vi "PulseDetectAndSwitch60.vi"(9 "Laser bits in":bool[](array[boolean])=[FALSE, FALSE, FALSE, FALSE, FALSE, FALSE, FALSE, FALSE, FALSE, FALSE, FALSE, FALSE, FALSE, FALSE, FALSE, FALSE, FALSE, FALSE, FALSE, FALSE, FALSE, FALSE, FALSE, FALSE, FALSE, FALSE, FALSE, FALSE, FALSE, FALSE, FALSE, FALSE, FALSE, FALSE, FALSE, FALSE, FALSE, FALSE, FALSE, FALSE, FALSE, FALSE, FALSE, FALSE, FALSE, FALSE, FALSE, FALSE, FALSE, FALSE, FALSE, FALSE, FALSE, FALSE, FALSE, FALSE, FALSE, FALSE, FALSE, FALSE], 10 "Last area":bool, 11 "Last laser bit in":bool) -> (1 "Area bits out":bool[](array[boolean]), 2 "New last area out":bool, 3 "New last laser bit out":bool)   [LabVIEW 2012]
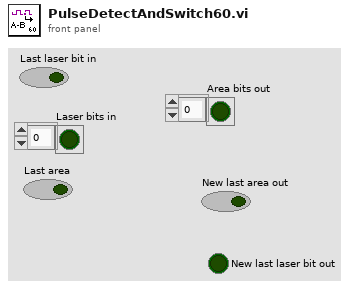
[diagram p1: front panel]
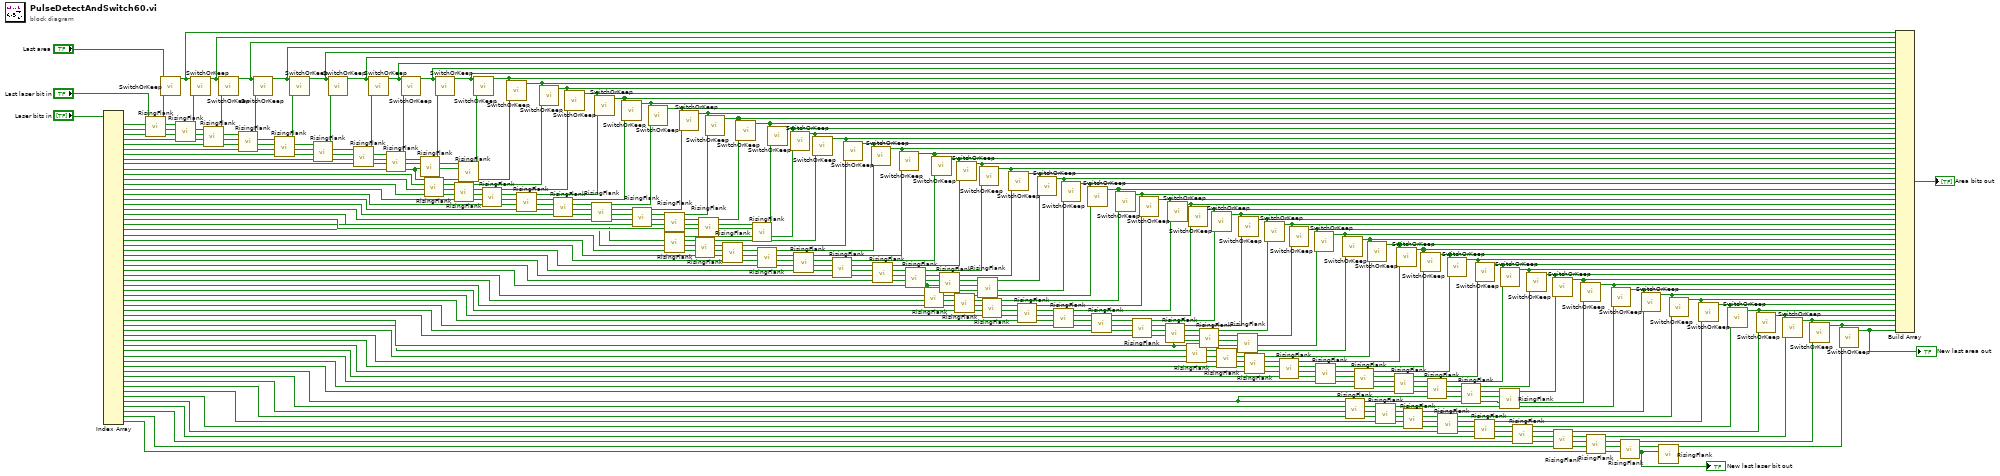
[diagram p0: block diagram]
diagram:
  n1 = Index Array(array="Laser bits in") -> (element #1=w182:bool, element #2=w181:bool, element #3=w180:bool, element #4=w179:bool, element #5=w178:bool, element #6=w177:bool, element #7=w176:bool, element #8=w175:bool, element #9=w174:bool, element #10=w152:bool, element #11=w151:bool, element #12=w150:bool, element #13=w149:bool, element #14=w148:bool, element #15=w147:bool, element #16=w146:bool, element #17=w145:bool, element #18=w144:bool, element #19=w143:bool, element #20=w142:bool, element #21=w141:bool, element #22=w140:bool, element #23=w139:bool, element #24=w138:bool, element #25=w1:bool, element #26=w137:bool, element #27=w136:bool, element #28=w135:bool, element #29=w134:bool, element #30=w133:bool, element #31=w132:bool, element #32=w131:bool, element #33=w130:bool, element #34=w129:bool, element #35=w2:bool, element #36=w128:bool, element #37=w127:bool, element #38=w126:bool, element #39=w125:bool, element #40=w124:bool, element #41=w123:bool, element #42=w3:bool, element #43=w122:bool, element #44=w121:bool, element #45=w120:bool, element #46=w119:bool, element #47=w118:bool, element #48=w4:bool, element #49=w117:bool, element #50=w116:bool, element #51=w115:bool, element #52=w114:bool, element #53=w113:bool, element #54=w112:bool, element #55=w111:bool, element #56=w110:bool, element #57=w109:bool, element #58=w108:bool, element #59=w107:bool, element #60=w106:bool)  [unwired: 60 in]
  "New last laser bit out" <- w106
  n2 = call "RisingFlank.vi"("2nd sample"=w182, "1st sample"="Last laser bit in") -> ("Rising flank?"=w172:bool)  [unwired: 7 in]
  n3 = call "SwitchOrKeep.vi"("Rising flank? in"=w172, "Last state in"="Last area") -> ("New state out"=w162:bool)  [unwired: 9 in]
  n4 = call "RisingFlank.vi"("2nd sample"=w181, "1st sample"=w182) -> ("Rising flank?"=w171:bool)  [unwired: 7 in]
  n5 = call "SwitchOrKeep.vi"("Rising flank? in"=w171, "Last state in"=w162) -> ("New state out"=w161:bool)  [unwired: 9 in]
  n6 = call "RisingFlank.vi"("2nd sample"=w180, "1st sample"=w181) -> ("Rising flank?"=w170:bool)  [unwired: 7 in]
  n7 = call "SwitchOrKeep.vi"("Rising flank? in"=w170, "Last state in"=w161) -> ("New state out"=w160:bool)  [unwired: 9 in]
  n8 = call "RisingFlank.vi"("2nd sample"=w179, "1st sample"=w180) -> ("Rising flank?"=w169:bool)  [unwired: 7 in]
  n9 = call "SwitchOrKeep.vi"("Rising flank? in"=w169, "Last state in"=w160) -> ("New state out"=w159:bool)  [unwired: 9 in]
  n10 = call "RisingFlank.vi"("2nd sample"=w178, "1st sample"=w179) -> ("Rising flank?"=w168:bool)  [unwired: 7 in]
  n11 = call "SwitchOrKeep.vi"("Rising flank? in"=w168, "Last state in"=w159) -> ("New state out"=w158:bool)  [unwired: 9 in]
  n12 = call "RisingFlank.vi"("2nd sample"=w177, "1st sample"=w178) -> ("Rising flank?"=w167:bool)  [unwired: 7 in]
  n13 = call "SwitchOrKeep.vi"("Rising flank? in"=w167, "Last state in"=w158) -> ("New state out"=w157:bool)  [unwired: 9 in]
  n14 = call "RisingFlank.vi"("2nd sample"=w176, "1st sample"=w177) -> ("Rising flank?"=w166:bool)  [unwired: 7 in]
  n15 = call "SwitchOrKeep.vi"("Rising flank? in"=w166, "Last state in"=w157) -> ("New state out"=w156:bool)  [unwired: 9 in]
  n16 = call "RisingFlank.vi"("2nd sample"=w175, "1st sample"=w176) -> ("Rising flank?"=w165:bool)  [unwired: 7 in]
  n17 = call "SwitchOrKeep.vi"("Rising flank? in"=w165, "Last state in"=w156) -> ("New state out"=w155:bool)  [unwired: 9 in]
  n18 = call "RisingFlank.vi"("2nd sample"=w174, "1st sample"=w175) -> ("Rising flank?"=w164:bool)  [unwired: 7 in]
  n19 = call "RisingFlank.vi"("2nd sample"=w151, "1st sample"=w152) -> ("Rising flank?"=w104:bool)  [unwired: 7 in]
  n20 = call "SwitchOrKeep.vi"("Rising flank? in"=w164, "Last state in"=w155) -> ("New state out"=w154:bool)  [unwired: 9 in]
  n21 = call "RisingFlank.vi"("2nd sample"=w150, "1st sample"=w151) -> ("Rising flank?"=w102:bool)  [unwired: 7 in]
  n22 = call "RisingFlank.vi"("2nd sample"=w152, "1st sample"=w174) -> ("Rising flank?"=w163:bool)  [unwired: 7 in]
  n23 = call "SwitchOrKeep.vi"("Rising flank? in"=w163, "Last state in"=w154) -> ("New state out"=w105:bool)  [unwired: 9 in]
  n24 = call "RisingFlank.vi"("2nd sample"=w149, "1st sample"=w150) -> ("Rising flank?"=w100:bool)  [unwired: 7 in]
  n25 = call "SwitchOrKeep.vi"("Rising flank? in"=w104, "Last state in"=w105) -> ("New state out"=w103:bool)  [unwired: 9 in]
  n26 = call "RisingFlank.vi"("2nd sample"=w148, "1st sample"=w149) -> ("Rising flank?"=w98:bool)  [unwired: 7 in]
  n27 = call "SwitchOrKeep.vi"("Rising flank? in"=w102, "Last state in"=w103) -> ("New state out"=w101:bool)  [unwired: 9 in]
  n28 = call "RisingFlank.vi"("2nd sample"=w147, "1st sample"=w148) -> ("Rising flank?"=w96:bool)  [unwired: 7 in]
  n29 = call "SwitchOrKeep.vi"("Rising flank? in"=w100, "Last state in"=w101) -> ("New state out"=w99:bool)  [unwired: 9 in]
  n30 = call "RisingFlank.vi"("2nd sample"=w146, "1st sample"=w147) -> ("Rising flank?"=w94:bool)  [unwired: 7 in]
  n31 = call "SwitchOrKeep.vi"("Rising flank? in"=w98, "Last state in"=w99) -> ("New state out"=w97:bool)  [unwired: 9 in]
  n32 = call "SwitchOrKeep.vi"("Rising flank? in"=w96, "Last state in"=w97) -> ("New state out"=w95:bool)  [unwired: 9 in]
  n33 = call "RisingFlank.vi"("2nd sample"=w145, "1st sample"=w146) -> ("Rising flank?"=w92:bool)  [unwired: 7 in]
  n34 = call "SwitchOrKeep.vi"("Rising flank? in"=w94, "Last state in"=w95) -> ("New state out"=w93:bool)  [unwired: 9 in]
  n35 = call "RisingFlank.vi"("2nd sample"=w144, "1st sample"=w145) -> ("Rising flank?"=w91:bool)  [unwired: 7 in]
  n36 = call "RisingFlank.vi"("2nd sample"=w141, "1st sample"=w142) -> ("Rising flank?"=w84:bool)  [unwired: 7 in]
  n37 = call "SwitchOrKeep.vi"("Rising flank? in"=w92, "Last state in"=w93) -> ("New state out"=w90:bool)  [unwired: 9 in]
  n38 = call "RisingFlank.vi"("2nd sample"=w140, "1st sample"=w141) -> ("Rising flank?"=w82:bool)  [unwired: 7 in]
  n39 = call "RisingFlank.vi"("2nd sample"=w143, "1st sample"=w144) -> ("Rising flank?"=w88:bool)  [unwired: 7 in]
  n40 = call "SwitchOrKeep.vi"("Rising flank? in"=w91, "Last state in"=w90) -> ("New state out"=w89:bool)  [unwired: 9 in]
  n41 = call "RisingFlank.vi"("2nd sample"=w139, "1st sample"=w140) -> ("Rising flank?"=w80:bool)  [unwired: 7 in]
  n42 = call "SwitchOrKeep.vi"("Rising flank? in"=w88, "Last state in"=w89) -> ("New state out"=w87:bool)  [unwired: 9 in]
  n43 = call "RisingFlank.vi"("2nd sample"=w142, "1st sample"=w143) -> ("Rising flank?"=w86:bool)  [unwired: 7 in]
  n44 = call "RisingFlank.vi"("2nd sample"=w138, "1st sample"=w139) -> ("Rising flank?"=w78:bool)  [unwired: 7 in]
  n45 = call "SwitchOrKeep.vi"("Rising flank? in"=w86, "Last state in"=w87) -> ("New state out"=w85:bool)  [unwired: 9 in]
  n46 = call "SwitchOrKeep.vi"("Rising flank? in"=w84, "Last state in"=w85) -> ("New state out"=w83:bool)  [unwired: 9 in]
  n47 = call "RisingFlank.vi"("2nd sample"=w1, "1st sample"=w138) -> ("Rising flank?"=w76:bool)  [unwired: 7 in]
  n48 = call "SwitchOrKeep.vi"("Rising flank? in"=w82, "Last state in"=w83) -> ("New state out"=w81:bool)  [unwired: 9 in]
  n49 = call "RisingFlank.vi"("2nd sample"=w137, "1st sample"=w1) -> ("Rising flank?"=w74:bool)  [unwired: 7 in]
  n50 = call "SwitchOrKeep.vi"("Rising flank? in"=w80, "Last state in"=w81) -> ("New state out"=w79:bool)  [unwired: 9 in]
  n51 = call "SwitchOrKeep.vi"("Rising flank? in"=w78, "Last state in"=w79) -> ("New state out"=w77:bool)  [unwired: 9 in]
  n52 = call "RisingFlank.vi"("2nd sample"=w136, "1st sample"=w137) -> ("Rising flank?"=w72:bool)  [unwired: 7 in]
  n53 = call "SwitchOrKeep.vi"("Rising flank? in"=w76, "Last state in"=w77) -> ("New state out"=w75:bool)  [unwired: 9 in]
  n54 = call "RisingFlank.vi"("2nd sample"=w135, "1st sample"=w136) -> ("Rising flank?"=w70:bool)  [unwired: 7 in]
  n55 = call "RisingFlank.vi"("2nd sample"=w132, "1st sample"=w133) -> ("Rising flank?"=w64:bool)  [unwired: 7 in]
  n56 = call "SwitchOrKeep.vi"("Rising flank? in"=w74, "Last state in"=w75) -> ("New state out"=w73:bool)  [unwired: 9 in]
  n57 = call "RisingFlank.vi"("2nd sample"=w134, "1st sample"=w135) -> ("Rising flank?"=w68:bool)  [unwired: 7 in]
  n58 = call "RisingFlank.vi"("2nd sample"=w131, "1st sample"=w132) -> ("Rising flank?"=w62:bool)  [unwired: 7 in]
  n59 = call "SwitchOrKeep.vi"("Rising flank? in"=w72, "Last state in"=w73) -> ("New state out"=w71:bool)  [unwired: 9 in]
  n60 = call "RisingFlank.vi"("2nd sample"=w133, "1st sample"=w134) -> ("Rising flank?"=w66:bool)  [unwired: 7 in]
  n61 = call "SwitchOrKeep.vi"("Rising flank? in"=w70, "Last state in"=w71) -> ("New state out"=w69:bool)  [unwired: 9 in]
  n62 = call "RisingFlank.vi"("2nd sample"=w130, "1st sample"=w131) -> ("Rising flank?"=w60:bool)  [unwired: 7 in]
  n63 = call "SwitchOrKeep.vi"("Rising flank? in"=w68, "Last state in"=w69) -> ("New state out"=w67:bool)  [unwired: 9 in]
  n64 = call "RisingFlank.vi"("2nd sample"=w129, "1st sample"=w130) -> ("Rising flank?"=w58:bool)  [unwired: 7 in]
  n65 = call "SwitchOrKeep.vi"("Rising flank? in"=w66, "Last state in"=w67) -> ("New state out"=w65:bool)  [unwired: 9 in]
  n66 = call "RisingFlank.vi"("2nd sample"=w2, "1st sample"=w129) -> ("Rising flank?"=w56:bool)  [unwired: 7 in]
  n67 = call "SwitchOrKeep.vi"("Rising flank? in"=w64, "Last state in"=w65) -> ("New state out"=w63:bool)  [unwired: 9 in]
  n68 = call "SwitchOrKeep.vi"("Rising flank? in"=w62, "Last state in"=w63) -> ("New state out"=w61:bool)  [unwired: 9 in]
  n69 = call "RisingFlank.vi"("2nd sample"=w128, "1st sample"=w2) -> ("Rising flank?"=w55:bool)  [unwired: 7 in]
  n70 = call "SwitchOrKeep.vi"("Rising flank? in"=w60, "Last state in"=w61) -> ("New state out"=w59:bool)  [unwired: 9 in]
  n71 = call "RisingFlank.vi"("2nd sample"=w127, "1st sample"=w128) -> ("Rising flank?"=w54:bool)  [unwired: 7 in]
  n72 = call "SwitchOrKeep.vi"("Rising flank? in"=w58, "Last state in"=w59) -> ("New state out"=w57:bool)  [unwired: 9 in]
  n73 = call "RisingFlank.vi"("2nd sample"=w126, "1st sample"=w127) -> ("Rising flank?"=w53:bool)  [unwired: 7 in]
  n74 = call "SwitchOrKeep.vi"("Rising flank? in"=w56, "Last state in"=w57) -> ("New state out"=w52:bool)  [unwired: 9 in]
  n75 = call "RisingFlank.vi"("2nd sample"=w123, "1st sample"=w124) -> ("Rising flank?"=w35:bool)  [unwired: 7 in]
  n76 = call "SwitchOrKeep.vi"("Rising flank? in"=w55, "Last state in"=w52) -> ("New state out"=w51:bool)  [unwired: 9 in]
  n77 = call "RisingFlank.vi"("2nd sample"=w125, "1st sample"=w126) -> ("Rising flank?"=w49:bool)  [unwired: 7 in]
  n78 = call "SwitchOrKeep.vi"("Rising flank? in"=w54, "Last state in"=w51) -> ("New state out"=w50:bool)  [unwired: 9 in]
  n79 = call "RisingFlank.vi"("2nd sample"=w3, "1st sample"=w123) -> ("Rising flank?"=w34:bool)  [unwired: 7 in]
  n80 = call "RisingFlank.vi"("2nd sample"=w124, "1st sample"=w125) -> ("Rising flank?"=w46:bool)  [unwired: 7 in]
  n81 = call "SwitchOrKeep.vi"("Rising flank? in"=w53, "Last state in"=w50) -> ("New state out"=w48:bool)  [unwired: 9 in]
  n82 = call "RisingFlank.vi"("2nd sample"=w122, "1st sample"=w3) -> ("Rising flank?"=w33:bool)  [unwired: 7 in]
  n83 = call "SwitchOrKeep.vi"("Rising flank? in"=w49, "Last state in"=w48) -> ("New state out"=w47:bool)  [unwired: 9 in]
  n84 = call "RisingFlank.vi"("2nd sample"=w121, "1st sample"=w122) -> ("Rising flank?"=w32:bool)  [unwired: 7 in]
  n85 = call "SwitchOrKeep.vi"("Rising flank? in"=w46, "Last state in"=w47) -> ("New state out"=w45:bool)  [unwired: 9 in]
  n86 = call "SwitchOrKeep.vi"("Rising flank? in"=w35, "Last state in"=w45) -> ("New state out"=w44:bool)  [unwired: 9 in]
  n87 = call "RisingFlank.vi"("2nd sample"=w120, "1st sample"=w121) -> ("Rising flank?"=w31:bool)  [unwired: 7 in]
  n88 = call "SwitchOrKeep.vi"("Rising flank? in"=w34, "Last state in"=w44) -> ("New state out"=w43:bool)  [unwired: 9 in]
  n89 = call "RisingFlank.vi"("2nd sample"=w115, "1st sample"=w116) -> ("Rising flank?"=w15:bool)  [unwired: 7 in]
  n90 = call "RisingFlank.vi"("2nd sample"=w119, "1st sample"=w120) -> ("Rising flank?"=w30:bool)  [unwired: 7 in]
  n91 = call "SwitchOrKeep.vi"("Rising flank? in"=w33, "Last state in"=w43) -> ("New state out"=w42:bool)  [unwired: 9 in]
  n92 = call "RisingFlank.vi"("2nd sample"=w114, "1st sample"=w115) -> ("Rising flank?"=w14:bool)  [unwired: 7 in]
  n93 = call "RisingFlank.vi"("2nd sample"=w118, "1st sample"=w119) -> ("Rising flank?"=w29:bool)  [unwired: 7 in]
  n94 = call "SwitchOrKeep.vi"("Rising flank? in"=w32, "Last state in"=w42) -> ("New state out"=w41:bool)  [unwired: 9 in]
  n95 = call "RisingFlank.vi"("2nd sample"=w113, "1st sample"=w114) -> ("Rising flank?"=w13:bool)  [unwired: 7 in]
  n96 = call "SwitchOrKeep.vi"("Rising flank? in"=w31, "Last state in"=w41) -> ("New state out"=w40:bool)  [unwired: 9 in]
  n97 = call "RisingFlank.vi"("2nd sample"=w4, "1st sample"=w118) -> ("Rising flank?"=w28:bool)  [unwired: 7 in]
  n98 = call "RisingFlank.vi"("2nd sample"=w112, "1st sample"=w113) -> ("Rising flank?"=w12:bool)  [unwired: 7 in]
  n99 = call "SwitchOrKeep.vi"("Rising flank? in"=w30, "Last state in"=w40) -> ("New state out"=w39:bool)  [unwired: 9 in]
  n100 = call "RisingFlank.vi"("2nd sample"=w117, "1st sample"=w4) -> ("Rising flank?"=w27:bool)  [unwired: 7 in]
  n101 = call "RisingFlank.vi"("2nd sample"=w111, "1st sample"=w112) -> ("Rising flank?"=w11:bool)  [unwired: 7 in]
  n102 = call "SwitchOrKeep.vi"("Rising flank? in"=w29, "Last state in"=w39) -> ("New state out"=w38:bool)  [unwired: 9 in]
  n103 = call "RisingFlank.vi"("2nd sample"=w116, "1st sample"=w117) -> ("Rising flank?"=w26:bool)  [unwired: 7 in]
  n104 = call "SwitchOrKeep.vi"("Rising flank? in"=w28, "Last state in"=w38) -> ("New state out"=w37:bool)  [unwired: 9 in]
  n105 = call "RisingFlank.vi"("2nd sample"=w110, "1st sample"=w111) -> ("Rising flank?"=w10:bool)  [unwired: 7 in]
  n106 = call "SwitchOrKeep.vi"("Rising flank? in"=w27, "Last state in"=w37) -> ("New state out"=w36:bool)  [unwired: 9 in]
  n107 = call "SwitchOrKeep.vi"("Rising flank? in"=w26, "Last state in"=w36) -> ("New state out"=w25:bool)  [unwired: 9 in]
  n108 = call "RisingFlank.vi"("2nd sample"=w109, "1st sample"=w110) -> ("Rising flank?"=w9:bool)  [unwired: 7 in]
  n109 = call "SwitchOrKeep.vi"("Rising flank? in"=w15, "Last state in"=w25) -> ("New state out"=w24:bool)  [unwired: 9 in]
  n110 = call "RisingFlank.vi"("2nd sample"=w108, "1st sample"=w109) -> ("Rising flank?"=w8:bool)  [unwired: 7 in]
  n111 = call "SwitchOrKeep.vi"("Rising flank? in"=w14, "Last state in"=w24) -> ("New state out"=w23:bool)  [unwired: 9 in]
  n112 = call "RisingFlank.vi"("2nd sample"=w107, "1st sample"=w108) -> ("Rising flank?"=w7:bool)  [unwired: 7 in]
  n113 = call "SwitchOrKeep.vi"("Rising flank? in"=w13, "Last state in"=w23) -> ("New state out"=w22:bool)  [unwired: 9 in]
  n114 = call "RisingFlank.vi"("2nd sample"=w106, "1st sample"=w107) -> ("Rising flank?"=w6:bool)  [unwired: 7 in]
  n115 = call "SwitchOrKeep.vi"("Rising flank? in"=w12, "Last state in"=w22) -> ("New state out"=w21:bool)  [unwired: 9 in]
  n116 = call "SwitchOrKeep.vi"("Rising flank? in"=w11, "Last state in"=w21) -> ("New state out"=w20:bool)  [unwired: 9 in]
  n117 = call "SwitchOrKeep.vi"("Rising flank? in"=w10, "Last state in"=w20) -> ("New state out"=w19:bool)  [unwired: 9 in]
  n118 = call "SwitchOrKeep.vi"("Rising flank? in"=w9, "Last state in"=w19) -> ("New state out"=w18:bool)  [unwired: 9 in]
  n119 = call "SwitchOrKeep.vi"("Rising flank? in"=w8, "Last state in"=w18) -> ("New state out"=w17:bool)  [unwired: 9 in]
  n120 = call "SwitchOrKeep.vi"("Rising flank? in"=w7, "Last state in"=w17) -> ("New state out"=w16:bool)  [unwired: 9 in]
  n121 = call "SwitchOrKeep.vi"("Rising flank? in"=w6, "Last state in"=w16) -> ("New state out"=w5:bool)  [unwired: 9 in]
  "New last area out" <- w5
  n122 = Build Array(w162, w161, w160, w159, w158, w157, w156, w155, w154, w105, w103, w101, w99, w97, w95, w93, w90, w89, w87, w85, w83, w81, w79, w77, w75, w73, w71, w69, w67, w65, w63, w61, w59, w57, w52, w51, w50, w48, w47, w45, w44, w43, w42, w41, w40, w39, w38, w37, w36, w25, w24, w23, w22, w21, w20, w19, w18, w17, w16, w5) -> (→"Area bits out":bool[])
